vi "sub_frame_to_packets2.vi"(9 "packet size":i32=1600, 10 "Cluster":cluster{i32, "Data String":string}) -> (2 "packets":cluster{i16[]}[](array[cluster]))   [LabVIEW 2014]
panel:
  out "length":i32
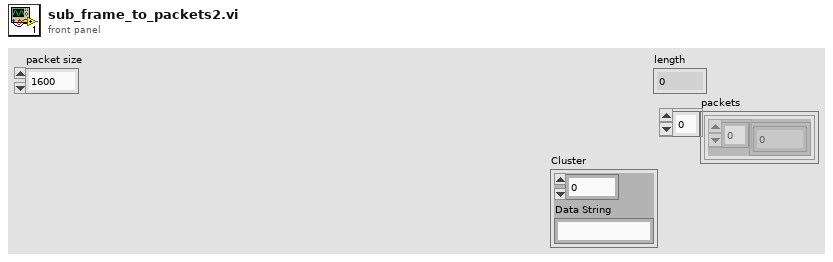
[diagram p1: front panel]
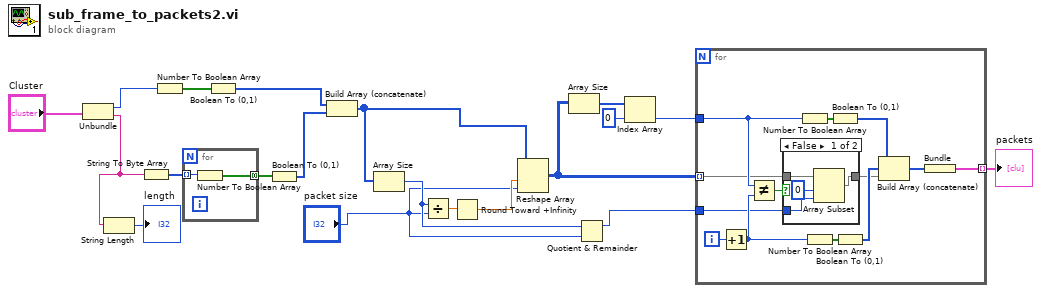
[diagram p0: block diagram]
diagram:
  n1 = Unbundle("Cluster") -> (w16:i32, "Data String"=w6:string)
  n2 = String Length(string=w6) -> (length=→"length":i32)
  n3 = String To Byte Array(string=w6) -> (unsigned byte array=w19:u8[])
  n4 = Number To Boolean Array(number=w16) -> (Boolean array=w17:bool[])
  n5 = for {
    tunnel: w19 -> [w22] mode=indexing
    tunnel: [w21] -> w18 mode=concatenating
    n6 = Number To Boolean Array(number=w22) -> (Boolean array=w21:bool[])
  }
  n7 = Boolean To (0,1)(Boolean=w17) -> (0, 1=w14:i16[])
  n8 = Boolean To (0,1)(Boolean=w18) -> (0, 1=w15:i16[])
  n9 = Build Array (concatenate)(w14, w15) -> (w11:i16[])
  n10 = Array Size(array=w11) -> (size(s)=w4:i32)
  n11 = Divide(x=w4, y="packet size") -> (x/y=w13:dbl)
  n12 = Round Toward +Infinity(x=w13) -> (ceil(x): smallest int >= x=w12:dbl)
  n13 = Reshape Array(w11, w12, "packet size") -> (w10:i16[][])
  n14 = Array Size(array=w10) -> (size(s)=w9:i32[])
  n15 = Quotient & Remainder(x=w4, y="packet size") -> (x-y*floor(x/y)=w2:i32)  [unwired: 1 out]
  n16 = Index Array(array=w9, index=0) -> (element=w8:i32)
  n17 = for {
    tunnel: w10 -> [w28] mode=indexing
    tunnel: w8 -> [w34]
    tunnel: w2 -> [w25]
    tunnel: [w23] -> w1 mode=indexing
    i -> [w35]
    n18 = Increment(x=w35) -> (x+1=w33:i32)
    n19 = Not Equal?(x=w34, y=w33) -> (x != y?=w27:bool)
    n20 = case shown="False" w27 {
      tunnel: w28 -> [w39 w40]
      tunnel: [w38 w40] -> w26
      tunnel: w25 -> [w37 _]
      frame False {
        n21 = Array Subset(array=w39, index=0, length=w37) -> (w38:i16[])
      }
      frame True {
      }
    }
    n22 = Number To Boolean Array(number=w34) -> (Boolean array=w30:bool[])
    n23 = Number To Boolean Array(number=w33) -> (Boolean array=w32:bool[])
    n24 = Boolean To (0,1)(Boolean=w30) -> (0, 1=w29:i16[])
    n25 = Boolean To (0,1)(Boolean=w32) -> (0, 1=w31:i16[])
    n26 = Build Array (concatenate)(w29, w31, w26) -> (w24:i16[])
    n27 = Bundle(w24) -> (w23:cluster{i16[]})  [unwired: 1 in]
  }
  "packets" <- w1
